vi "AR.Drone MAIN.vi"() -> ()   [LabVIEW 2014]
uses:
  Resources/Others/Control cluster.ctl
  <vilib>/LVH/AR Drone Toolkit/Decode NavData/Typedefs/NavData Demo.ctl
  Resources/Global.vi
  Kinect Extention/Kinect Global.vi
  <vilib>/LVH/AR Drone Toolkit/AR Drone.lvlib
panel:
  in  "Tab Control 3":enum32{"Flight Control"}(tab)
  in  "Manual":bool=TRUE
  in  "Switch control":bool
  in  "Enable Kinect Extention":bool
  in  "Tab Control 2":enum32{"Setup", "Debug&Test Info", "NavData"}(tab)
  in  "Enable Video":bool
  in  "Enable Controller Setup":bool
  in  "Reset OCR":bool
  in  "Secondary VI":u16(ring)=1 items=["Auto Hovering with Position Prediction.vi", "Simple Video.vi", "Circle detection.vi", "OCR Control.vi"]
  in  "Setup Parameters":T1={"Drone IP address"="192.168.1.1", "Home IP address"="192.168.1.2", "Flight Mode"=enum."INDOOR MODE", "Mounted Hull"=enum."INDOOR HULL", "Video Camera"=0, "Max Altitude (m)"=3.0, "Max Pitch and Roll Angle (deg)"=8.0, "Max Vertical Speed (m/s)"=0.7, "Max Yaw Speed (deg/s)"=100.0} {"Video Camera" items=["Bottom Camera"=1, "Front Camera"=0, "Front in Bottom"=3, "Bottom in Front"=2]}
  in  "Adjustments (affects Secondary VIs)":cluster{"Sensitivity":dbl, "Null Zone":dbl}={"Sensitivity"=1.0, "Null Zone"=1.0} {"Null Zone" scale=0.0..2.0; "Sensitivity" scale=0.0..2.0}
  in  "Enable Kinect Setup":bool
  out "Succesful Controller Setup":bool
  out "Succesful Drone Setup":bool
  in  "Control loop wait (ms)":u32=25
  out "Control loop Refesh Rate (ms)":u32
  in  "Video acquisition wait (ms)":u32=30
  out "Loop error":errorcluster
  out "Setup error":errorcluster
  out "Loop error (Ctr & Nav)":bool
  in  "Clear errors":bool
  out "Video procesing Refresh Rate (ms)":i32
  out "NavData Out":T2={"control state"=enum."INIT", "battery percentage"=100, "pitch (deg)"=0.0, "roll (deg)"=0.0, "yaw (deg)"=0.0, "altitude (cm)"=0, "vx (cm/s)?"=0.0, "vy (cm/s)?"=0.0, "vz (cm/s)?"=0.0, "detection cam type"=3}
  out "Battery Remaining":dbl(slide)=100.0 scale=0.0..100.0
  out "Hover (H)":bool
  out "Control Cluster":T3 {"Yaw Speed" scale=-1.0..1.0; "Vertical Speed" scale=-1.0..1.0; "Pitch" scale=-1.0..1.0; "Roll" scale=-1.0..1.0}
  out "Take off/Land (T)":bool
  in  "Tab Control":T4(tab)
  out "Raw":picture
  in  "Take photo":bool
  out "Generated path":path
  out "Error creating image":errorcluster
  out "Grayscale":T5(plugin-control)
  out "B&W":T5(plugin-control)
  in  "Calibrate Pitch":bool
  out "3D Picture":refnum<vi>(3d-picture)
  in  "stop":bool
  in  "Emergency Landing":bool
  # "Select Manual/Auto Control (based on Secondary VI)"
  # "Keyboard/Controller input"
  # "Enable Kinect gestuires (BETA)"
  # "(1 is default)"
  # "FOR ADVANCED USERS ONLY!"
  # "Not recommended!!!"
  # "This ignores the errors but does NOT eliminate them!"
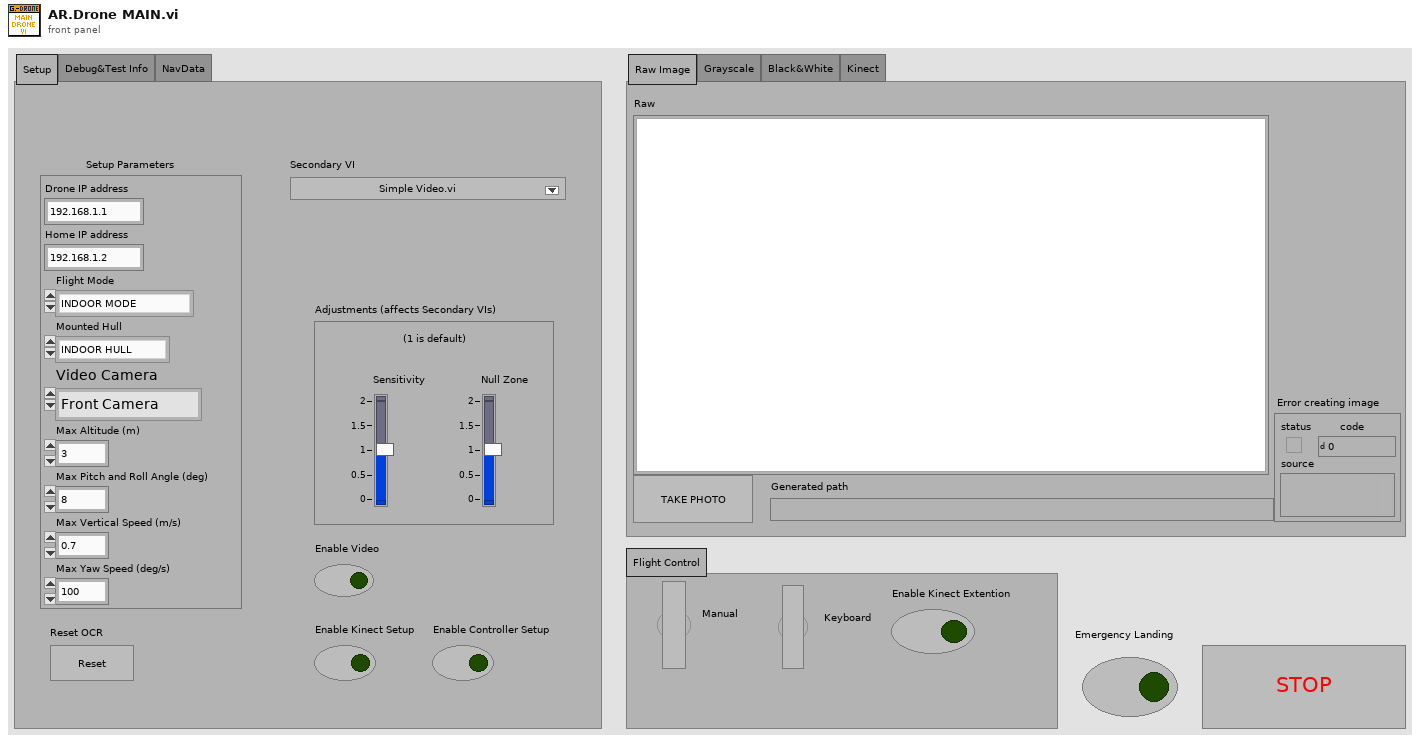
[diagram p1: front panel]
types:
  T1 = cluster{"Drone IP address":string, "Home IP address":string, "Flight Mode":enum8{"OUTDOOR MODE", "INDOOR MODE"}, "Mounted Hull":enum8{"OUTDOOR HULL", "INDOOR HULL"}, "Video Camera":u8, "Max Altitude (m)":sgl, "Max Pitch and Roll Angle (deg)":sgl, "Max Vertical Speed (m/s)":sgl, "Max Yaw Speed (deg/s)":sgl}
  T2 = typedef "AR Drone.lvlib/NavData Demo.ctl" = cluster{"control state":enum32{"DEFAULT", "INIT", "LANDING", "FLYING", "HOVERING", "TEST", "TRANS_TAKEOFF", "TRANS_GOTOFIX", "TRANS_LANDING"}, "battery percentage":u32, "pitch (deg)":sgl, "roll (deg)":sgl, "yaw (deg)":sgl, "altitude (cm)":u32, "vx (cm/s)?":sgl, "vy (cm/s)?":sgl, "vz (cm/s)?":sgl, "detection cam type":u32}
  T3 = typedef "Control cluster.ctl" = cluster{"Roll":sgl, "Pitch":sgl, "Vertical Speed":sgl, "Yaw Speed":sgl}
  T4 = enum32{"Raw Image", "Grayscale", "Black&White", "Kinect"}
  T5 = typedef "IMAQ Image.ctl" = refnum<image>
  T6 = typedef "imagedata.ctl" = cluster{"image type":i32, "image depth":i32, "image":u8[], "mask":u8[], "colors":u32[], "Rectangle":cluster{"left":i16, "top":i16, "right":i16, "bottom":i16}}
  T7 = typedef "AR Drone.lvlib/AR Drone Resource.ctl" = cluster{"UDP Control Connection":refnum<k16>, "UDP NavData Connection":refnum<k16>, "UDP Video Connection (Drone 1.0)":refnum<k16>, "TCP Video Connection (Drone 2.0)":refnum<k5>, "TCP Control Port Connection":refnum<k5>, "Drone IP address":string, "Drone Command Port":u16, "Drone NavData Port":u16, "Drone Vid Stream Port":u16, "Drone TCP Control Port":u16, "Home IP address":string, "Home Command Port":u16, "Home NavData Port":u16, "Home Vid Stream Port":u16, "Drone Version":i32, "Drone Index":i32, "Command Sequence":i32}
  T8 = cluster{"Roll":dbl, "Pitch":dbl, "Vertical Speed":dbl, "Yaw Speed":dbl}
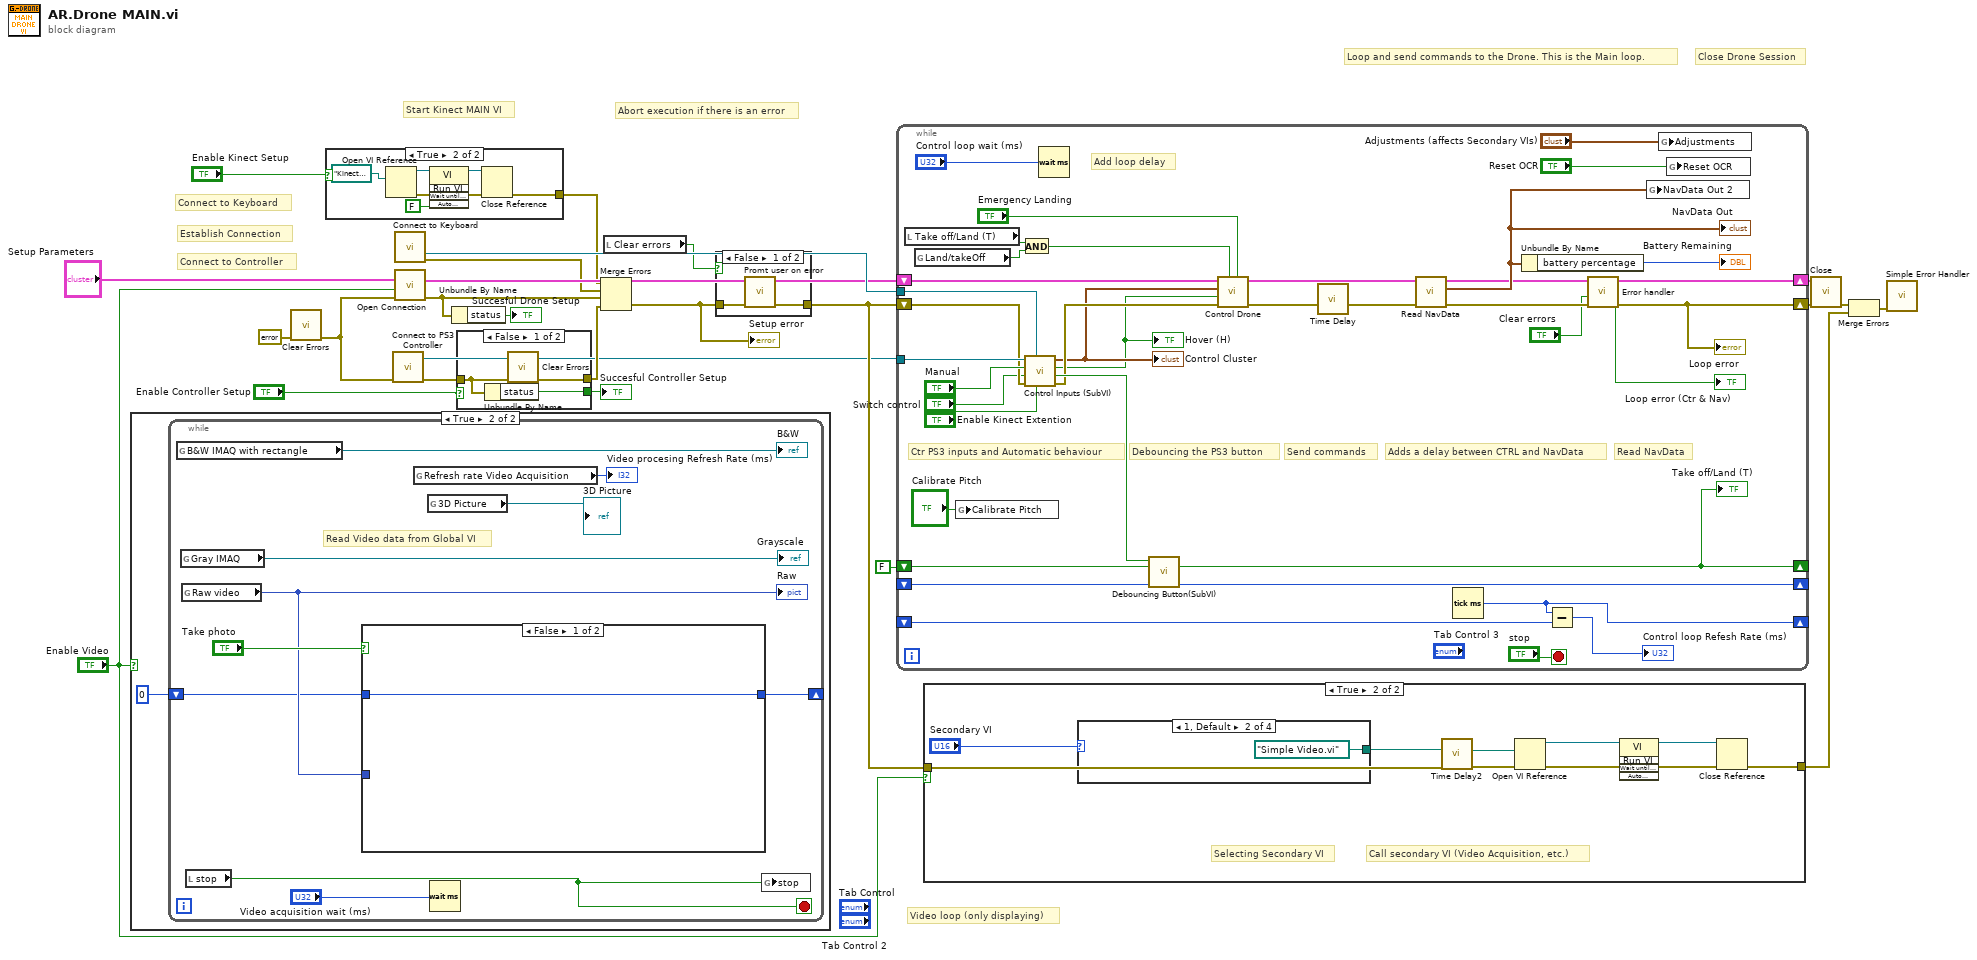
[diagram p0: block diagram]
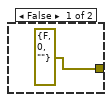
[diagram p2: hidden frame]
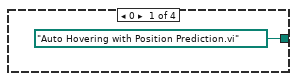
[diagram p4: hidden frame]
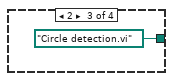
[diagram p5: hidden frame]
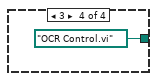
[diagram p6: hidden frame]
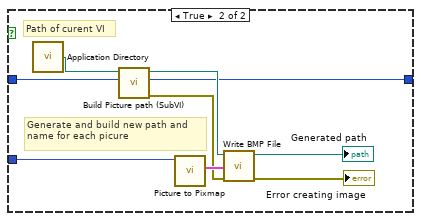
[diagram p8: hidden frame]
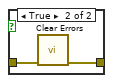
[diagram p9: hidden frame]
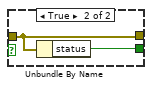
[diagram p10: hidden frame]
diagram:
  # "Start Kinect MAIN VI"
  # "Video loop (only displaying)"
  # "Connect to Keyboard"
  # "Connect to Controller"
  # "Abort execution if there is an error"
  # "Establish Connection"
  # "Close Drone Session"
  # "Loop and send commands to the Drone. This is the Main loop."
  n1 = case shown="True" "Enable Video" {
    frame False {
    }
    frame True {
      n2 = while {
        shift-right: [w29] -> _
        shift-left: 0 -> [w30]
        stop <- w36 stop-if-true
        # "Read Video data from Global VI"
        n3 = global read "Global.vi" "B&W IMAQ with rectangle"() -> (→"B&W":T5)
        n4 = global read "Global.vi" "Gray IMAQ"() -> (→"Grayscale":T5)
        n5 = global read "Global.vi" "Raw video"() -> (w31:picture)
        "Raw" <- w31
        n6 = local read "stop"() -> (w36:bool)
        n7 = case shown="False" "Take photo" {
          tunnel: w31 -> [_ w44]
          tunnel: w30 -> [w37 w42]
          tunnel: [w37 w41] -> w29
          frame False {
          }
          frame True {
            # "Generate and build new path and name for each picure"
            # "Path of curent VI"
            n8 = call <vilib>:"Application Directory.vi"() -> ("Application Directory"=w40:path)
            n9 = call "Build Picture path (SubVI).vi"("Numeric in"=w42, "Application Directory"=w40) -> ("Error Out"=w38:errorcluster, "Numeric out"=w41:i32, "Path"=w45:path)  [unwired: 7 in]
            n10 = call <vilib>:"Picture to Pixmap.vi"("picture"=w44) -> ("image data"=w46:T6)  [unwired: 9 in, 1 out]
            n11 = call <vilib>:"Write BMP File.vi"("error in (no error)"=w38, "image data"=w46, "path to BMP file"=w45) -> ("error out"=→"Error creating image":errorcluster, "path"=→"Generated path":path)  [unwired: 7 in]
          }
        }
        n12 = global read "Global.vi" "Refresh rate Video Acquisition"() -> (→"Video procesing Refresh Rate (ms)":i64)
        n13 = global read "Kinect Global.vi" "3D Picture"() -> (→"3D Picture":refnum<vi>)
        n14 = Wait (ms)(milliseconds to wait="Video acquisition wait (ms)") -> ()  [unwired: 1 out]
        n15 = global write "Global.vi" "stop"(w36) -> ()
      }
    }
  }
  n16 = call <vilib>:"Clear Errors.vi"("error in (no error)"=errorcluster {"status"=FALSE, "code"=0, "source"=""}) -> ("error out"=w11:errorcluster)  [unwired: 5 in, 1 out]
  n17 = case shown="True" "Enable Kinect Setup" {
    tunnel: [errorcluster {"status"=FALSE, "code"=0, "source"=""} ("error out") w50] -> w2
    frame False {
    }
    frame True {
      n18 = Open VI Reference(vi path=path "Kinect Extention/Kinect MAIN.vi") -> (vi reference=w52:refnum<vi>, error out=w51:errorcluster)  [unwired: 5 in]
      n19 = invoke on="Invoke Node" class="VI" method="Run VI"(reference=w52, error in=w51, "Wait until done"=FALSE ("Wait Until Done")) -> (reference out=w53:refnum<vi>, error out=w54:errorcluster)  [unwired: 2 in, 3 out]
      n20 = Close Reference(reference=w53, error in (no error)=w54) -> (error out=w50:errorcluster)
    }
  }
  n21 = call "Connect to PS3 Controller.vi"("error in (no error)"=w11) -> ("error out"=w9:errorcluster, "device ID 2"=w7:refnum<k1>)  [unwired: 8 in]
  n22 = call "Connect to Keyboard.vi"() -> ("device ID"=w16:refnum<k1>, "error out"=w13:errorcluster)  [unwired: 13 in, 1 out]
  n23 = call "Open Connection.vi"("error in (no error)"=w11, "Init Video?"="Enable Video", "Setup Parameters"="Setup Parameters") -> ("error out"=w14:errorcluster, "AR Drone Resource"=w15:T7)  [unwired: 7 in]
  n24 = Unbundle By Name(w14) -> ("status"=→"Succesful Drone Setup":bool)
  n25 = case shown="False" "Enable Controller Setup" {
    tunnel: w9 -> [w56 w59]
    tunnel: [w57 w59] -> w8
    tunnel: [w55 w58] -> w6
    frame False {
      n26 = Unbundle By Name(w56) -> ("status"=w55:bool)
      n27 = call <vilib>:"Clear Errors.vi"("error in (no error)"=w56) -> ("error out"=w57:errorcluster)  [unwired: 5 in, 1 out]
    }
    frame True {
      n28 = Unbundle By Name(w59) -> ("status"=w58:bool)
    }
  }
  "Succesful Controller Setup" <- w6
  n29 = Merge Errors(w2, w13, w14, w8) -> (w3:errorcluster)
  "Setup error" <- w3
  n30 = local read "Clear errors"() -> (w5:bool)
  n31 = case shown="False" w5 {
    tunnel: w3 -> [w61 w63]
    tunnel: [w60 w62] -> w12
    frame False {
      n32 = call "Promt user on error.vi"("error in (no error)"=w61) -> ("error out"=w60:errorcluster)  [unwired: 10 in]
    }
    frame True {
      n33 = call <vilib>:"Clear Errors.vi"("error in (no error)"=w63) -> ("error out"=w62:errorcluster)  [unwired: 5 in, 1 out]
    }
  }
  n34 = while {
    shift-right: [w83] -> w25
    shift-left: w15 -> [w99]
    shift-right: [w67] -> w23
    shift-left: w12 -> [w79]
    shift-right: [w76] -> _
    shift-left: _ -> [w95]
    shift-right: [w92] -> _
    shift-left: FALSE -> [w93]
    shift-right: [w91] -> _
    shift-left: _ -> [w90]
    tunnel: w7 -> [w85]
    tunnel: w16 -> [w69]
    stop <- "stop" stop-if-true
    # "Add loop delay"
    # "Ctr PS3 inputs and Automatic behaviour"
    # "Read NavData"
    # "Send commands"
    # "Debouncing the PS3 button"
    # "Adds a delay between CTRL and NavData"
    n35 = local read "Take off/Land (T)"() -> (w74:bool)
    n36 = global read "Global.vi" "Land/takeOff"() -> (w75:bool)
    n37 = global write "Kinect Global.vi" "Calibrate Pitch"("Calibrate Pitch") -> ()
    n38 = And(x=w74, y=w75) -> (x .and. y?=w86:bool)
    n39 = call "Control Inputs (SubVI).vi"("Enable Kinect Extention"="Enable Kinect Extention", "Keyboard ID"=w69, "error in (no error)"=w79, "Switch control"="Switch control", "Manual"="Manual", "Controller ID"=w85) -> ("error out"=w78:errorcluster, "Land/Take off"=w94:bool, "Hover Out"=w73:bool, "Control cluster"=w77:T8)  [unwired: 2 in]
    "Control Cluster" <- w77
    "Hover (H)" <- w73
    n40 = Wait (ms)(milliseconds to wait="Control loop wait (ms)") -> ()  [unwired: 1 out]
    n41 = call "Debouncing Button(SubVI).vi"("millisecond timer value in"=w90, "Boolean in"=w93, "Land/Take off"=w94) -> ("millisecond timer value out"=w91:u32, "Boolean out"=w92:bool)  [unwired: 7 in]
    "Take off/Land (T)" <- w92
    n42 = call <vilib>:"Control Drone.vi"("Emergency Landing"="Emergency Landing", "Takeoff/Land"=w86, "error in (no error)"=w78, "Hover"=w73, "Control Cluster"=w77, "AR Drone Resource"=w99) -> ("error out"=w81:errorcluster, "AR Drone Resource Out"=w98:T7)  [unwired: 4 in]
    n43 = call "Time Delay"("error in (no error)"=w81) -> ("error out"=w82:errorcluster)  [unwired: 10 in]
    n44 = call <vilib>:"Read NavData.vi"("error in (no error)"=w82, "AR Drone Resource"=w98) -> ("error out"=w68:errorcluster, "NavData Out"=w87:T2, "AR Drone Resource Out"=w83:T7)  [unwired: 7 in]
    "NavData Out" <- w87
    n45 = Tick Count (ms)() -> (millisecond timer value=w76:u32)
    n46 = Unbundle By Name(w87) -> ("battery percentage"=→"Battery Remaining":u32)
    n47 = Subtract(x=w76, y=w95) -> (x-y=→"Control loop Refesh Rate (ms)":u32)
    n48 = call "Error handler.vi"("error in (no error)"=w68, "Clear errors"="Clear errors") -> ("error out"=w67:errorcluster, "status"=→"Loop error (Ctr & Nav)":bool)  [unwired: 8 in]
    "Loop error" <- w67
    n49 = global write "Global.vi" "NavData Out 2"(w87) -> ()
    n50 = global write "Global.vi" "Adjustments"("Adjustments (affects Secondary VIs)") -> ()
    n51 = global write "Global.vi" "Reset OCR"("Reset OCR") -> ()
  }
  n52 = case shown="True" "Enable Video" {
    tunnel: [w101 w106] -> w19
    tunnel: w12 -> [w101 w102]
    frame False {
    }
    frame True {
      # "Selecting Secondary VI"
      # "Call secondary VI (Video Acquisition, etc.)"
      n53 = case shown="1, Default" "Secondary VI" {
        tunnel: [path "Auto Hovering with Position Prediction.vi" ("Video Acquisition VI path") path "Simple Video.vi" ("Video Acquisition VI path") path "Circle detection.vi" ("Video Acquisition VI path") path "OCR Control.vi" ("Video Acquisition VI path")] -> w105
        frame 0 {
        }
        frame 1, Default {
        }
        frame 2 {
        }
        frame 3 {
        }
      }
      n54 = call "Time Delay2"("error in (no error)"=w102) -> ("error out"=w109:errorcluster)  [unwired: 10 in]
      n55 = Open VI Reference(vi path=w105, error in (no error)=w109) -> (vi reference=w104:refnum<vi>, error out=w103:errorcluster)  [unwired: 4 in]
      n56 = invoke class="VI" method="Run VI"(reference=w104, error in=w103) -> (reference out=w108:refnum<vi>, error out=w110:errorcluster)  [unwired: 3 in, 3 out]
      n57 = Close Reference(reference=w108, error in (no error)=w110) -> (error out=w106:errorcluster)
    }
  }
  n58 = call <vilib>:"Close.vi"("error in (no error)"=w23, "AR Drone Resource"=w25) -> ("error out"=w20:errorcluster)  [unwired: 9 in]
  n59 = Merge Errors(w20, w19) -> (w22:errorcluster)
  n60 = call <vilib>:"Simple Error Handler.vi"("error in (no error)"=w22) -> ()  [unwired: 4 in, 5 out]
